vi "设置延时.vi"(8 "error in (no error)":errorcluster caption="错误输入（无错误）", 11 "数字多用表接口 输入":refnum<class "数字多用表接口.lvclass">) -> (0 "error out":errorcluster caption="错误输出", 3 "数字多用表接口 输出":refnum<class "数字多用表接口.lvclass">)   [LabVIEW 2020, in "数字多用表接口.lvlib" / "数字多用表接口.lvclass"]
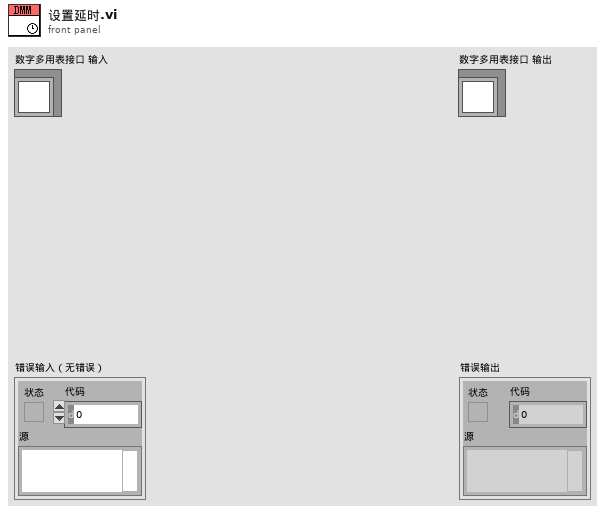
[diagram p1: front panel]
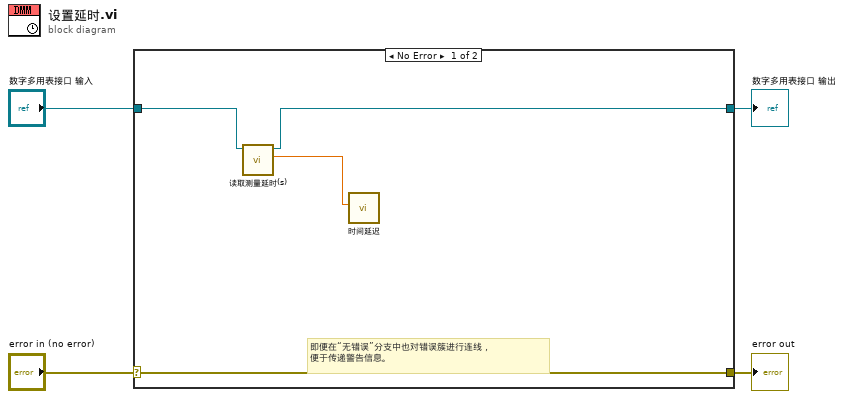
[diagram p0: block diagram]
diagram:
  n1 = case shown="No Error" "error in (no error)" {
    selector: "error in (no error)" -> [w8 w10]
    tunnel: [w8 w10] -> w3
    tunnel: [w6 w9] -> w1
    tunnel: "数字多用表接口 输入" -> [w7 w9]
    frame No Error {
      # "即便在“无错误”分支中也对错误簇进行连线，\n便于传递警告信息。"
      n2 = call "读取测量延时(s).vi"("数字多用表接口输入"=w7) -> ("测量延时(s)"=w5:dbl, "数字多用表接口输出"=w6:refnum<class "数字多用表接口.lvclass">)  [unwired: 8 in, 1 out]
      n3 = call "时间延迟"("Delay Time (s)"=w5) -> ()  [unwired: 10 in, 1 out]
    }
    frame Error {
    }
  }
  "error out" <- w3
  "数字多用表接口 输出" <- w1
